vi "PulseHistogram_OnlyLaser.vi"() -> ()   [LabVIEW 2012]
doc: "This example demonstrates how to generate and acquire data up to eight channels using an NI 6587 adapter module. It generates either a constant value or a digital count-up pattern on the first eight even, odd, upper, or lower numbered channels of the DDC connector, and then acquires that pattern on the first eight odd, even, lower, or upper (respectively) numbered channels of the DDC connector. The data is generated on one cycle of the single-cycle timed loop and acquired on the next cycle of the loop. To properly verify the waveforms in this example, you must connect the first eight channels to the other eight channels on the DDC connector. For example, if you choose the Even to Odd Channel Configuration, connect the even numbered channels to the odd numbered channels (DIO 0 -> DIO 1, DIO 2 -> DIO 3,...DIO 14 -> DIO 15).\nThis getting started example is intended for lower clock rates depending on your setup. For high speed applications, refer to the Serdes Channel or Serdes Connector examples."
uses:
  <vilib>/Platform/TimedLoop/XDataNode/timing_clust.ctl
  <vilib>/Platform/TimedLoop/XDataNode/nitl_modes.ctl
  <vilib>/Platform/TimedLoop/XDataNode/wakeup.ctl
  <vilib>/rvi/Emulation/niFpgaSctlEmulationRegisterWithScheduler.vi
  <vilib>/rvi/eio/common/nirviEmuTemplateMethod_errors.vi
  <vilib>/rvi/Emulation/niFpgaSctlEmulationScheduler.vi
  <vilib>/rvi/FIFO/Fifo_Resource/nirvififoEmulationSetSize.vi
  <vilib>/rvi/DataTransferAndStorage/Container/Common/niFpgaContainerGetUniqueNameForEmu.vi
  <vilib>/rvi/Emulation/niFpgaSctlEmulationFifoFullMgr.vi
  <vilib>/rvi/errors/niFpgaSetErrorForExecOnDevCompSimple.vi
  <vilib>/rvi/eio/common/nirviEmuReportErrorAndStop.vi
  <vilib>/rvi/interface/RandomDataEmulation/nirviRandomDataFPGAFIFO.vi
  <vilib>/rvi/interface/RandomDataEmulation/niFpgaRandomDataHandleErrors.vi
  <vilib>/rvi/Emulation/niFpgaSctlEmulationResourceMgr.vi
  <vilib>/Platform/TimedLoop/XDataNode/XDataNode.xnode
  <vilib>/eio/EIONode/EIONode.xnode
  <vilib>/rvi/DataTransferAndStorage/Container/XNode/niFpgaContainer.xnode
  <vilib>/rvi/FIFO/Fifo_Resource/nirvififoEmulationClear.vi
  <vilib>/rvi/FIFO/Fifo_Resource/nirvififoEmulationRead.vi
  <vilib>/rvi/interface/RandomDataEmulation/nirviRandomDataFpgaReadWriteTemplate.vi
  <vilib>/rvi/FIFO/Fifo_Resource/nirvififoEmulationWrite.vi
  <vilib>/Platform/TimedLoop/XDataNode/XDNodeRunTimeDep.lvlib
panel:
  in  "Acquire":bool
  in  "Acq_Reset":bool
  out "Interloop FIFO overflow":bool
  out "Onboard_Clock_Ready":bool
  in  "Onboard_Clock_Write_Data":u16
  in  "Onboard_Clock_Write":bool
  in  "Clock Source":u8(ring)=3 items=["Tristate"=0, "Sync Clock (PXIe only)"=2, "Adapter Module Onboard Clock"=3, "Strobe from Crosspoint Switch"=4, "Strobe Bypass"=5]
  in  "Xpoint_Switch_Write":bool
  out "Interloop FIFO timed out":bool
  out "ToHostLaserFIFO overflow":bool
  out "Xpoint_Switch_Ready":bool
  in  "Commit":bool
  # "PulseHistogram\nonly Laser channel"
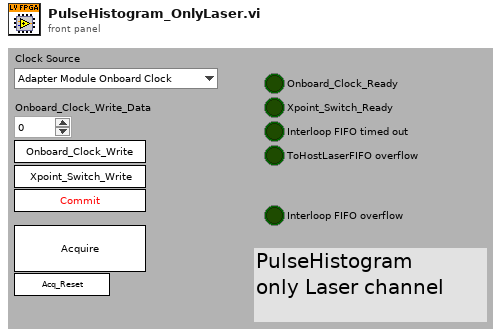
[diagram p1: front panel]
types:
  T1 = typedef "XDNodeRunTimeDep.lvlib/timing_clust.ctl" = cluster{"Expected End [f-1]":u64, "Actual End [f-1]":u64, "Finished Late? [f-1]":bool, "Expected End [i-1]":u64, "Actual End [i-1]":u64, "Finished Late? [i-1]":bool, "Expected Start [i]":u64, "Actual Start [i]":u64, "Expected Start [f]":u64, "Actual Start [f]":u64, "Source Name":string, "Structure Name":string, "Period":i64, "Deadline":i64, "Offset":i64, "Start":i64, "Priority":i32, "Timeout":i32, "Mode":T2, "Wakeup Reason":T3, "Error":errorcluster, "Source Type":string, "Secondary Source Type":string, "Global End Time":u64, "Global Start Time":u64, "Frame Duration":u64, "Iteration Duration":u64, "Assigned CPU":i32, "I/O Scan Engine Mode":u32}
  T2 = typedef "XDNodeRunTimeDep.lvlib/nitl_modes.ctl" = enum32{"No Change", "Process missed periods, maintain original phase", "Discard missed periods, maintain original phase", "Process missed periods, ignore original phase", "Discard missed periods, ignore original phase"}
  T3 = typedef "XDNodeRunTimeDep.lvlib/wakeup.ctl" = enum32{"Normal", "Aborted", "Asynchronous wakeup", "Timing source error", "Timed loop error", "Timeout"}
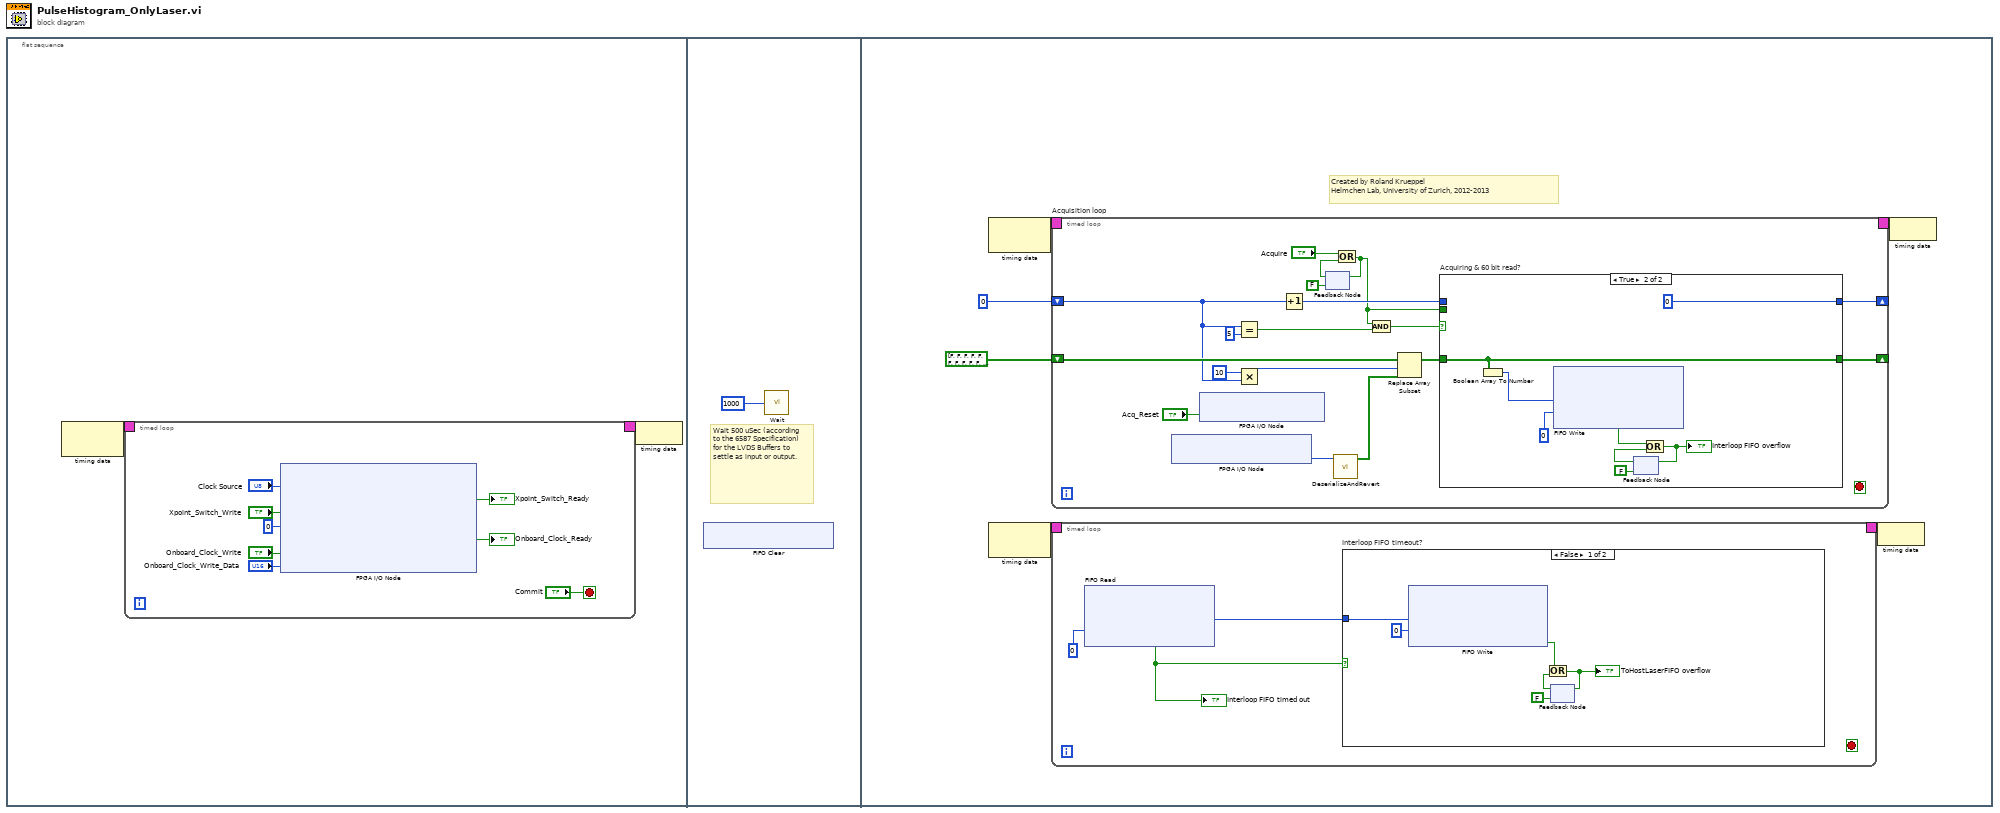
[diagram p0: block diagram]
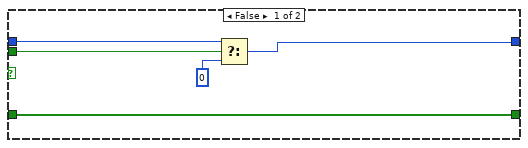
[diagram p2: hidden frame]
diagram:
  n1 = flat-sequence {
    frame #0 {
      n2 = node-c288() -> (w2:T1)  [unwired: 1 in]
      n3 = timed-loop {
        timing: w2 -> [_]
        timing-out: [_] -> w1
        stop <- "Commit" stop-if-true
        n4 = xnode "FPGA I/O Node"("IO Module\\Acq_IO_Clock_Source"="Clock Source", "IO Module\\Xpoint_Switch_Write"="Xpoint_Switch_Write", "IO Module\\LVDS_Data_Dir"=u16 0 ("IO Module\\LVDS_Data_Dir"), "IO Module\\Onboard_Clock_Write"="Onboard_Clock_Write", "IO Module\\Onboard_Clock_Write_Data"="Onboard_Clock_Write_Data") -> ("IO Module\\Xpoint_Switch_Ready"=→"Xpoint_Switch_Ready":bool, "IO Module\\Onboard_Clock_Ready"=→"Onboard_Clock_Ready":bool)  [unwired: 7 in, 7 out]
      }
      n5 = node-c288(w1) -> ()
    }
    frame #1 {
      # "Wait 500 uSec (according to the 6587 Specification) for the LVDS Buffers to settle as input or output."
      n6 = xnode ("FIFO Clear")() -> ()  [unwired: 1 in, 1 out]
      n7 = call "Wait"("Count(uSec)"=u32 1000 ("Wait (uSec)")) -> ()  [unwired: 1 out]
    }
    frame #2 {
      # "Created by Roland Krueppel\nHelmchen Lab, University of Zurich, 2012-2013"
      n8 = node-c288() -> (w19:T1)  [unwired: 1 in]
      n9 = node-c288() -> (w21:T1)  [unwired: 1 in]
      n10 = timed-loop "Acquisition loop" {
        timing: w19 -> [_]
        timing-out: [_] -> w18
        shift-right: [w35] -> _
        shift-left: bool[] [FALSE, FALSE, FALSE, FALSE, FALSE, FALSE, FALSE, FALSE, FALSE, FALSE, FALSE, FALSE, FALSE, FALSE, FALSE, FALSE, FALSE, FALSE, FALSE, FALSE, FALSE, FALSE, FALSE, FALSE, FALSE, FALSE, FALSE, FALSE, FALSE, FALSE, FALSE, FALSE, FALSE, FALSE, FALSE, FALSE, FALSE, FALSE, FALSE, FALSE, FALSE, FALSE, FALSE, FALSE, FALSE, FALSE, FALSE, FALSE, FALSE, FALSE, FALSE, FALSE, FALSE, FALSE, FALSE, FALSE, FALSE, FALSE, FALSE, FALSE] ("Boolean array") -> [w39]
        shift-right: [w34] -> _
        shift-left: 0 -> [w33]
        stop <- _ stop-if-true
        n11 = xnode "FPGA I/O Node"() -> ("IO Module\\LVDS_Ch0_Rd"=w30:u16)  [unwired: 1 in, 1 out]
        n12 = xnode "FPGA I/O Node"("IO Module\\Acq_Reset"="Acq_Reset") -> ()  [unwired: 1 in, 1 out]
        n13 = Equal?(x=w33, y=5) -> (x = y?=w28:bool)
        n14 = Multiply(x=10 ("y"), y=w33) -> (x*y=w32:i32)
        n15 = Increment(x=w33) -> (x+1=w31:i32)
        n16 = feedback #1(FALSE) -> (w24:bool)
        n17 = call "DeserializeAndRevert.vi"("U16 input"=w30) -> ("10bit output"=w29:bool[])  [unwired: 10 in]
        n18 = Or(x="Acquire", y=w24) -> (x .or. y?=w22:bool)
        n19 = feedback-in #1(w22) -> ()
        n20 = And(x=w22, y=w28) -> (x .and. y?=w27:bool)
        n21 = Replace Array Subset(array=w39, new element=w29, index=w32) -> (w36:bool[])
        n22 = case "Acquiring & 60 bit read?" shown="True" w27 {
          tunnel: w36 -> [w44 w51]
          tunnel: [w44 w51] -> w35
          tunnel: [w41 0] -> w34
          tunnel: w31 -> [w42 _]
          tunnel: w22 -> [w43 _]
          frame False {
            n23 = Select(t=w42, s=w43, f=0) -> (s? t:f=w41:i32)
          }
          frame True {
            n24 = Boolean Array To Number(Boolean array=w51) -> (number=w49:u64)
            n25 = xnode ("FIFO Write")("Element"=w49, "Timeout"=0) -> ("Timed Out?"=w48:bool)  [unwired: 1 in, 1 out]
            n26 = feedback #2(FALSE) -> (w46:bool)
            n27 = Or(x=w48, y=w46) -> (x .or. y?=w47:bool)
            "Interloop FIFO overflow" <- w47
            n28 = feedback-in #2(w47) -> ()
          }
        }
      }
      n29 = timed-loop {
        timing: w21 -> [_]
        timing-out: [_] -> w20
        stop <- _ stop-if-true
        n30 = xnode ("FIFO Read")("Timeout"=0) -> ("Element"=w58:u64, "Timed Out?"=w57:bool)  [unwired: 1 in, 1 out]
        "Interloop FIFO timed out" <- w57
        n31 = case "Interloop FIFO timeout?" shown="False" w57 {
          tunnel: w58 -> [w65 _]
          frame False {
            n32 = xnode ("FIFO Write")("Element"=w65, "Timeout"=0) -> ("Timed Out?"=w63:bool)  [unwired: 1 in, 1 out]
            n33 = feedback #3(FALSE) -> (w61:bool)
            n34 = Or(x=w63, y=w61) -> (x .or. y?=w62:bool)
            "ToHostLaserFIFO overflow" <- w62
            n35 = feedback-in #3(w62) -> ()
          }
          frame True {
          }
        }
      }
      n36 = node-c288(w20) -> ()
      n37 = node-c288(w18) -> ()
    }
  }
